vi "Pre Launch Init.vi"(11 "SDO Manager Worker in":refnum<class "Response Matcher.lvclass">) -> (0 "error out":errorcluster, 3 "SDO Manager Worker out":refnum<class "Response Matcher.lvclass">)   [LabVIEW 2020, in "CANopen.lvlib" / "SDO Manager.lvlib" / "Response Matcher.lvclass"]
doc: "<p>(<strong>Filename</strong>: <span class=\"dnl\">Actor Framework.lvlib:Actor.lvclass:Pre Launch Init.vi</span>)</p>\n<p>Defines behavior that occurs after the <a href=\"nihelplauncher://docs/csh?context=lvcore_lvcomm_af_launch_nested_actor\">Launch Nested Actor</a> method is invoked but before the actor's Actor Core method begins running.</p>\n<p>By default, this method does nothing. A descendant class may override it to define behavior.</p>"
uses:
  Response Matcher.lvclass
  Response Matcher.lvclass/Response Matcher.ctl
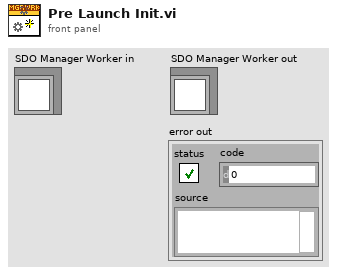
[diagram p1: front panel]
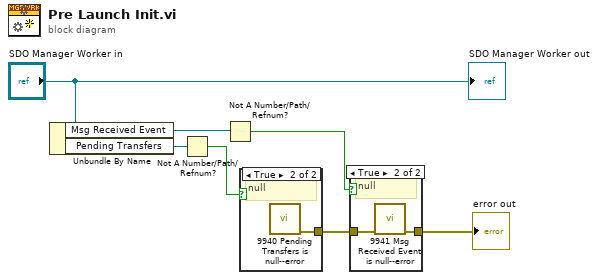
[diagram p0: block diagram]
diagram:
  n1 = Unbundle By Name("SDO Manager Worker in") -> ("Msg Received Event"=w6:refnum<user-event>, "Pending Transfers"=w5:refnum<data-value>)
  n2 = Not A Number/Path/Refnum?(number/path/refnum=w5) -> (NaN/Path/Refnum?=w4:bool)
  n3 = Not A Number/Path/Refnum?(number/path/refnum=w6) -> (NaN/Path/Refnum?=w3:bool)
  n4 = case shown="True" w4 {
    tunnel: [_ w8] -> w1
    frame False {
      # "not null"
    }
    frame True {
      # "null"
      n5 = call "9940 Pending Transfers is null--error.vi"() -> ("error out"=w8:errorcluster)  [unwired: 10 in, 1 out]
    }
  }
  n6 = case shown="True" w3 {
    tunnel: [w9 w10] -> w2
    tunnel: w1 -> [w9 w11]
    frame False {
      # "not null"
    }
    frame True {
      # "null"
      n7 = call "9941 Msg Received Event is null--error.vi"("error in"=w11) -> ("error out"=w10:errorcluster)  [unwired: 9 in, 1 out]
    }
  }
  "error out" <- w2
  "SDO Manager Worker out" <- "SDO Manager Worker in"
